vi "stripXmlFileHeader.vi"(8 "error in (no error)":errorcluster, 10 "XML File String":string) -> (0 "error out":errorcluster, 2 "XML File Document":string, 3 "XML File Header":string)   [LabVIEW 2011, in "EasyXMLTest.lvclass"]
uses:
  EasyXMLTest.lvclass
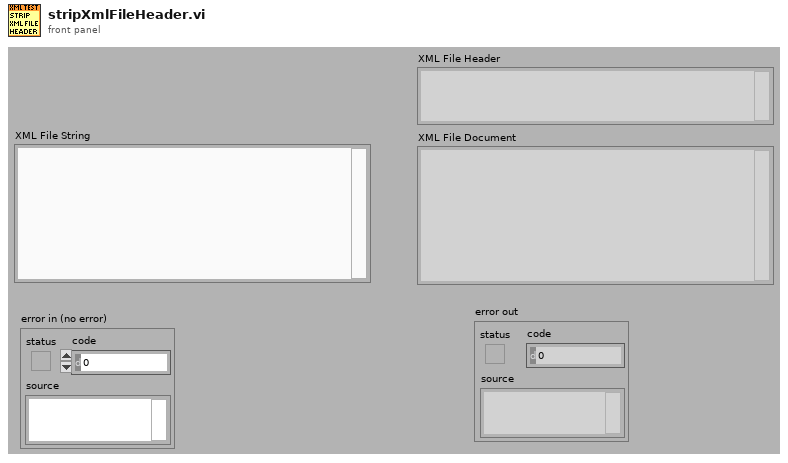
[diagram p1: front panel]
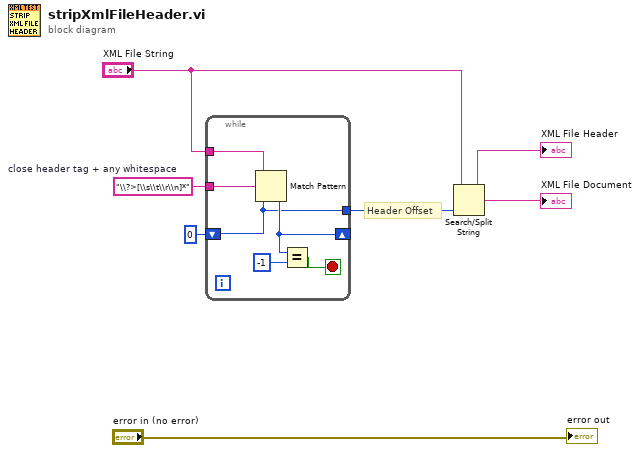
[diagram p0: block diagram]
diagram:
  w7 = "\\?>[\\s\\t\\r\\n]*"  # close header tag + any whitespace
  # "Header Offset"
  n1 = while {
    tunnel: w7 -> [w13]
    tunnel: "XML File String" -> [w8]
    shift-right: [w12] -> _
    shift-left: 0 ("offset past match") -> [w9]
    tunnel: [w9] -> w4
    stop <- w10 stop-if-true
    n2 = Match Pattern(string=w8, regular expression=w13, offset (0)=w9) -> (offset past match=w12:i32)  [unwired: 3 out]
    n3 = Equal?(x=w12, y=-1) -> (x = y?=w10:bool)
  }
  n4 = Search/Split String(string="XML File String", offset (0)=w4) -> (substring before match=→"XML File Header":string, match + rest of string=→"XML File Document":string)  [unwired: 1 in, 1 out]
  "error out" <- "error in (no error)"
